vi "Log Status Channels.vi"(10 "status channels refs":T1[](array[typedef]) format="%.0x", 11 "status channel offsets":u64[](array[numeric])) -> ()   [LabVIEW 2017, in "DSF Engine.lvlib" / "VeriStand DSF.lvclass"]
uses:
  VeriStand DSF.lvclass
  <vilib>/NI Veristand/Custom Device API/Custom Device Item Ref.ctl
  <vilib>/NI Veristand/Custom Device API/Custom Device API.lvlib
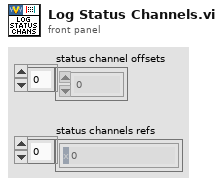
[diagram p1: front panel]
types:
  T1 = typedef "Custom Device API.lvlib/Custom Device Item Ref.ctl" = u64
  T2 = enum16{"open", "replace", "create", "open or create", "replace or create", "replace or create with confirmation"}
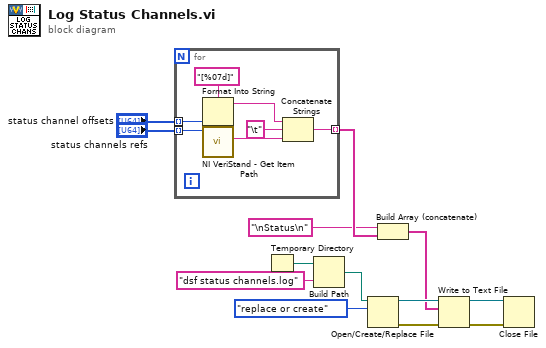
[diagram p0: block diagram]
diagram:
  n1 = for {
    tunnel: [w17] -> w11 mode=indexing
    tunnel: "status channel offsets" -> [w14] mode=indexing
    tunnel: "status channels refs" -> [w19] mode=indexing
    n2 = Format Into String(format string="[%07d]", w14) -> (resulting string=w15:string)  [unwired: 2 in, 1 out]
    n3 = call <vilib>:"NI VeriStand - Get Item Path.vi"("Item Ref in"=w19) -> ("Path"=w18:string)  [unwired: 7 in, 3 out]
    n4 = Concatenate Strings(w15, "\t" ("string"), w18) -> (w17:string)
  }
  n5 = Temporary Directory() -> (w9:path)
  n6 = Build Path(base path=w9, name or relative path="dsf status channels.log") -> (appended path=w7:path)
  n7 = Open/Create/Replace File(file path (use dialog)=w7, operation (0:open)=T2."replace or create") -> (refnum out=w6:refnum<file>, error out=w5:errorcluster)  [unwired: 4 in, 1 out]
  n8 = Build Array (concatenate)("\nStatus\n", w11) -> (w1:string[])
  n9 = Write to Text File(file (use dialog)=w6, text=w1, error in=w5) -> (refnum out=w3:refnum<file>, error out=w4:errorcluster)  [unwired: 1 in, 1 out]
  n10 = Close File(refnum=w3, error in=w4) -> ()  [unwired: 2 out]
